vi "Root.vi"(0 "f23":dbl, 1 "f24":dbl, 2 "f44":dbl) -> (20 "Root":dbl)   [LabVIEW 2014]
uses:
  <vilib>/Simulation/Implementation/Shared/SIMSCR Execution Mode.ctl
  <vilib>/Simulation/Scripting/Companion Diagram/SimConfigNode/SimParams.ctl
  <vilib>/Simulation/Scripting/Companion Diagram/SimConfigNode/_simSolvers.ctl
  <vilib>/Simulation/Param Hierarchy/Typedefs/SIMPH Param Control Actions.ctl
  <vilib>/Simulation/Implementation/Shared/NILVSim_ParamChanged.vi
  <vilib>/Simulation/Implementation/Shared/NILVSIM_BeginStep.vi
  <vilib>/Simulation/SignalArithmetic/Implementation/NILVSim Gain.llb/SIM Gain (scalar).vi
  <vilib>/Simulation/Implementation/Shared/NILVSim_Manager.vi
  <vilib>/Utility/error.llb/Clear Errors.vi
  <vilib>/Simulation/Implementation/Shared/NILVSim_FinalizeModel.vi
  <vilib>/Simulation/Implementation/Shared/SIM Unbundle Sim Info.vi
  <vilib>/Simulation/Implementation/Shared/SIMSH Read Queue.vi
  <vilib>/Simulation/Implementation/Shared/NILVSim_Initialize.vi
  <vilib>/Simulation/Utility/Implementation/NILVSim Get Time and IsAcceptedStep.vi
  <vilib>/Simulation/Implementation/Shared/NILVSim_GetModelError.vi
  <vilib>/Simulation/Implementation/Shared/SIM SimErrorHandler.vi
  <vilib>/Simulation/Implementation/Shared/SIM Bundle Sim Info.vi
  <vilib>/Simulation/Scripting/Companion Diagram/SimConfigNode/SimDog.xnode
  <vilib>/Simulation/Implementation/XNodeFramework/SimXNode/SimX.xnode
  <vilib>/Simulation/Implementation/Shared/NI_SIM_Implementation.lvlib
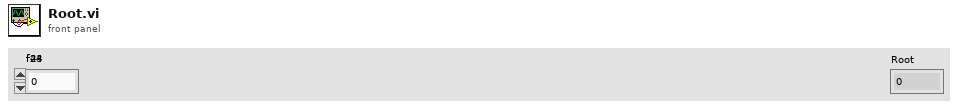
[diagram p1: front panel]
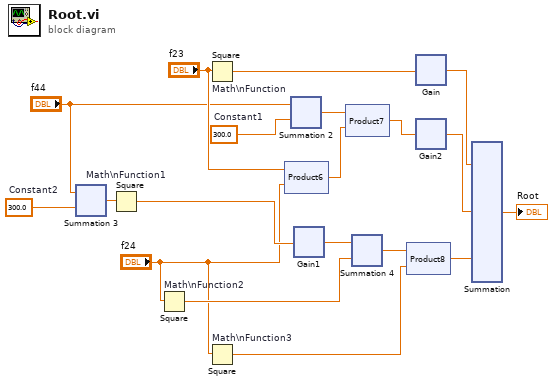
[diagram p0: block diagram]
diagram:
  w11 = 300.0  # Constant2
  w7 = 300.0  # Constant1
  n1 = xnode ("Summation 3")("Operand1"="f44", "Operand2"=w11) -> ("Result"=w19:dbl)
  n2 = Square "Math\\nFunction1"(x=w19) -> (x^2=w14:dbl)
  n3 = Square "Math\\nFunction2"(x="f24") -> (x^2=w6:dbl)
  n4 = Square "Math\\nFunction"(x="f23") -> (x^2=w15:dbl)
  n5 = Square "Math\\nFunction3"(x="f24") -> (x^2=w4:dbl)
  n6 = xnode "Product6"("Operand1"="f23", "Operand2"="f24") -> ("Result"=w5:dbl)
  n7 = xnode ("Summation 2")("Operand1"="f44", "Operand2"=w7) -> ("Result"=w17:dbl)
  n8 = xnode "Gain1"("input"=w14) -> ("output"=w18:dbl)  [unwired: 3 in]
  n9 = xnode "Product7"("Operand1"=w17, "Operand2"=w5) -> ("Result"=w9:dbl)
  n10 = xnode ("Summation 4")("Operand1"=w18, "Operand2"=w6) -> ("Result"=w13:dbl)
  n11 = xnode "Product8"("Operand1"=w13, "Operand2"=w4) -> ("Result"=w12:dbl)
  n12 = xnode "Gain"("input"=w15) -> ("output"=w16:dbl)  [unwired: 3 in]
  n13 = xnode "Gain2"("input"=w9) -> ("output"=w1:dbl)  [unwired: 3 in]
  n14 = xnode ("Summation")("Operand1"=w16, "Operand2"=w1, "Operand3"=w12) -> ("Result"=→"Root":dbl)
